vi "Begin.vi"(8 "error in":errorcluster) -> (0 "error out":errorcluster)   [LabVIEW 2015]
doc: "Called before other user functions, this VI is expected to open initial I/O refnums, load in file data, and do all program initialization. Notice that the <B>error out</B> terminal is simply used for data flow. Wiring it to other structures or subVIs ensures that this VI runs first."
uses:
  <vilib>/Rock Robotics/SystemInterfaces/DIO/FPGA_DIOPWMChannel.ctl
  <vilib>/Rock Robotics/WPI/SafetyOutput/WPI_SafetyOutputConfigMenu.ctl
  <vilib>/Rock Robotics/WPI/DriverStation/WPI_DriverStationRobotMode2.ctl
  <vilib>/Rock Robotics/WPI/Joystick/WPI_JoystickDeviceEnum.ctl
  <vilib>/Rock Robotics/WPI/Solenoid/WPI_SolenoidChannel.ctl
  <vilib>/Rock Robotics/SystemInterfaces/spilib/spi_bus.ctl
  <vilib>/Rock Robotics/SystemInterfaces/DIO/FPGA_DIOChannel.ctl
  <vilib>/Rock Robotics/WPI/RobotDrive/WPI_RobotDriveOpen2MotorWithVictor.vi
  Robot Global Data.vi
  <vilib>/Rock Robotics/Network Tables/NT Write String Array.vi
  <vilib>/Rock Robotics/WPI/MotorControl/WPI_MotorControlOpen Talon.vi
  <vilib>/Rock Robotics/WPI/Solenoid/WPI_SolenoidOpenDouble.vi
  <vilib>/Rock Robotics/WPI/Gyro/WPI_GyroXRS450_SPI_Open.vi
  <vilib>/Rock Robotics/WPI/MotorControl/WPI_MotorControlOpen Victor.vi
  <vilib>/Rock Robotics/WPI/Accelerometer/InternalAccelerometer/WPI_AccelerometerInternalOpen.vi
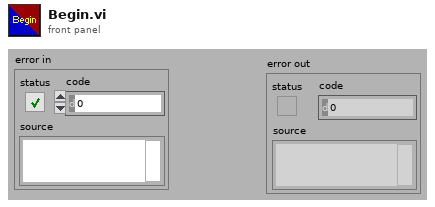
[diagram p1: front panel]
types:
  T1 = typedef "WPI_JoystickDeviceEnum.ctl" = enum16{"USB 0", "USB 1", "USB 2", "USB 3", "USB 4", "USB 5"}
  T2 = typedef "FPGA_DIOChannel.ctl" = enum8{"DIO 0", "DIO 1", "DIO 2", "DIO 3", "DIO 4", "DIO 5", "DIO 6", "DIO 7", "DIO 8", "DIO 9", "DIO MXP 0", "DIO MXP 1", "DIO MXP 2", "DIO MXP 3", "DIO MXP 4", "DIO MXP 5", "DIO MXP 6", "DIO MXP 7", "DIO MXP 8", "DIO MXP 9", "DIO MXP 10", "DIO MXP 11", "DIO MXP 12", "DIO MXP 13", "DIO MXP 14", "DIO MXP 15", "Invalid"}
  T3 = typedef "FPGA_DIOPWMChannel.ctl" = enum8{"PWM 0", "PWM 1", "PWM 2", "PWM 3", "PWM 4", "PWM 5", "PWM 6", "PWM 7", "PWM 8", "PWM 9", "PWM MXP 0", "PWM MXP 1", "PWM MXP 2", "PWM MXP 3", "PWM MXP 4", "PWM MXP 5", "PWM MXP 6", "PWM MXP 7", "PWM MXP 8", "PWM MXP 9", "Invalid"}
  T4 = typedef "WPI_SolenoidChannel.ctl" = enum8{"Solenoid 0", "Solenoid 1", "Solenoid 2", "Solenoid 3", "Solenoid 4", "Solenoid 5", "Solenoid 6", "Solenoid 7", "Invalid"}
  T5 = typedef "spi_bus.ctl" = enum16{"SPI On-Board, CS0", "SPI On-Board, CS1", "SPI On-Board, CS2", "SPI On-Board, CS3", "SPI MXP", "Invalid"}
  T6 = typedef "WPI_DriverStationRobotMode2.ctl" = enum16{"Autonomous Disabled", "Autonomous Enabled", "Teleop Disabled", "Teleop Enabled", "Disconnected", "Finish", "Test Disabled", "Test Enabled", "Emergency Stopped"}
  T7 = typedef "WPI_SafetyOutputConfigMenu.ctl" = enum16{"Enable", "Disable"}
  T8 = typedef "WPI_MotorControlDeviceRef.ctl" = cluster{"DeviceStatus":errorcluster, "Type":T9, "PWM":cluster{"PWM Channel":T3, "DeadBand":T10}, "CAN":cluster{"Device Number":u8, "Control Mode":T11, "Semaphore":T12, "Max Vout":dbl, "TalonSRX Control Mode":T13}, "Invert":bool}
  T9 = typedef "WPI_MotorControlType.ctl" = enum16{"PWM", "CAN", "CANTalonSRX"}
  T10 = typedef "WPI_PWMDeadband.ctl" = cluster{"Name":string, "maxPositivePwm":i32, "minPositivePwm":i32, "centerPwm":i32, "maxNegativePwm":i32, "minNegativePwm":i32, "angularRange":u16}
  T11 = typedef "WPI_CANJaguar_ControlMode.ctl" = enum8{"Percent VBus", "Current", "Speed", "Position", "Voltage"}
  T12 = typedef "Semaphore RefNum" = refnum<k1>
  T13 = typedef "WPI_CANTalonSRX_APIControlMode.ctl" = enum8{"Percent VBus", "Speed", "Position", "Slave", "Unchanged / Invalid", "Voltage Compensation", "Current", "Motion Profile"}
  T14 = typedef "WPI_JoystickDevRef.ctl" = cluster{"Device":T1}
  T15 = typedef "WPI_DigitalInputDevRef.ctl" = cluster{"DevStatus":errorcluster, "DIO Channel":T2}
  T16 = typedef "WPI_SolenoidDevRef.ctl" = cluster{"DevStatus":errorcluster, "Pneumatics Control Module":u8, "Forward Solenoid Channel":T4, "Reverse Solenoid Channel":T4}
  T17 = typedef "WPI_RobotDriveDevRef.ctl" = cluster{"DevStatus":errorcluster, "Motors[]":T8[], "Square Inputs":bool, "Max Output":dbl}
  T18 = typedef "WPI_GyroDevRef.ctl" = cluster{"DevStatus":errorcluster, "Analog Channel":T19, "Offset":dbl, "Gain (VoltsPerDegree/Second)":dbl, "Gyro Type":enum16{"Analog", "XRS450"}, "Handle":i32, "SPI Bus":T5, "Device Found":bool, "Sample Rate":dbl, "Calibrate On Open":bool}
  T19 = typedef "FPGA_AIChannel.ctl" = enum8{"AI 0", "AI 1", "AI 2", "AI 3", "AI MXP 0", "AI MXP 1", "AI MXP 2", "AI MXP 3", "Invalid"}
  T20 = typedef "WPI_AccelerometerDevRef.ctl" = cluster{"DevStatus":errorcluster, "Scaling":T21, "Analog Channels":T22, "I2C Bus":T23, "SPI Bus":T5, "Accel Range":T24, "ADXL Axes":T25, "Handle":i32, "Device Address":u8, "Accel Type":enum16{"Analog", "ADXL345 I2C", "ADXL345 SPI", "Internal", "ADXL362 SPI"}}
  T21 = typedef "WPI_AccelerometerScaling.ctl" = cluster{"Gain (VoltsPerG)":dbl, "Center Voltage":dbl}
  T22 = typedef "WPI_AccelerometerAnalogChannels.ctl" = cluster{"X-Axis":T19, "Y-Axis":T19, "Z-Axis":T19}
  T23 = typedef "i2c_bus.ctl" = enum16{"I2C On-Board", "I2C MXP", "Invalid"}
  T24 = typedef "ADXL345 Range.ctl" = u8
  T25 = typedef "WPI_AccelerometerADXL345 Axes.ctl" = cluster{"X-Axis":bool, "Y-Axis":bool, "Z-Axis":bool}
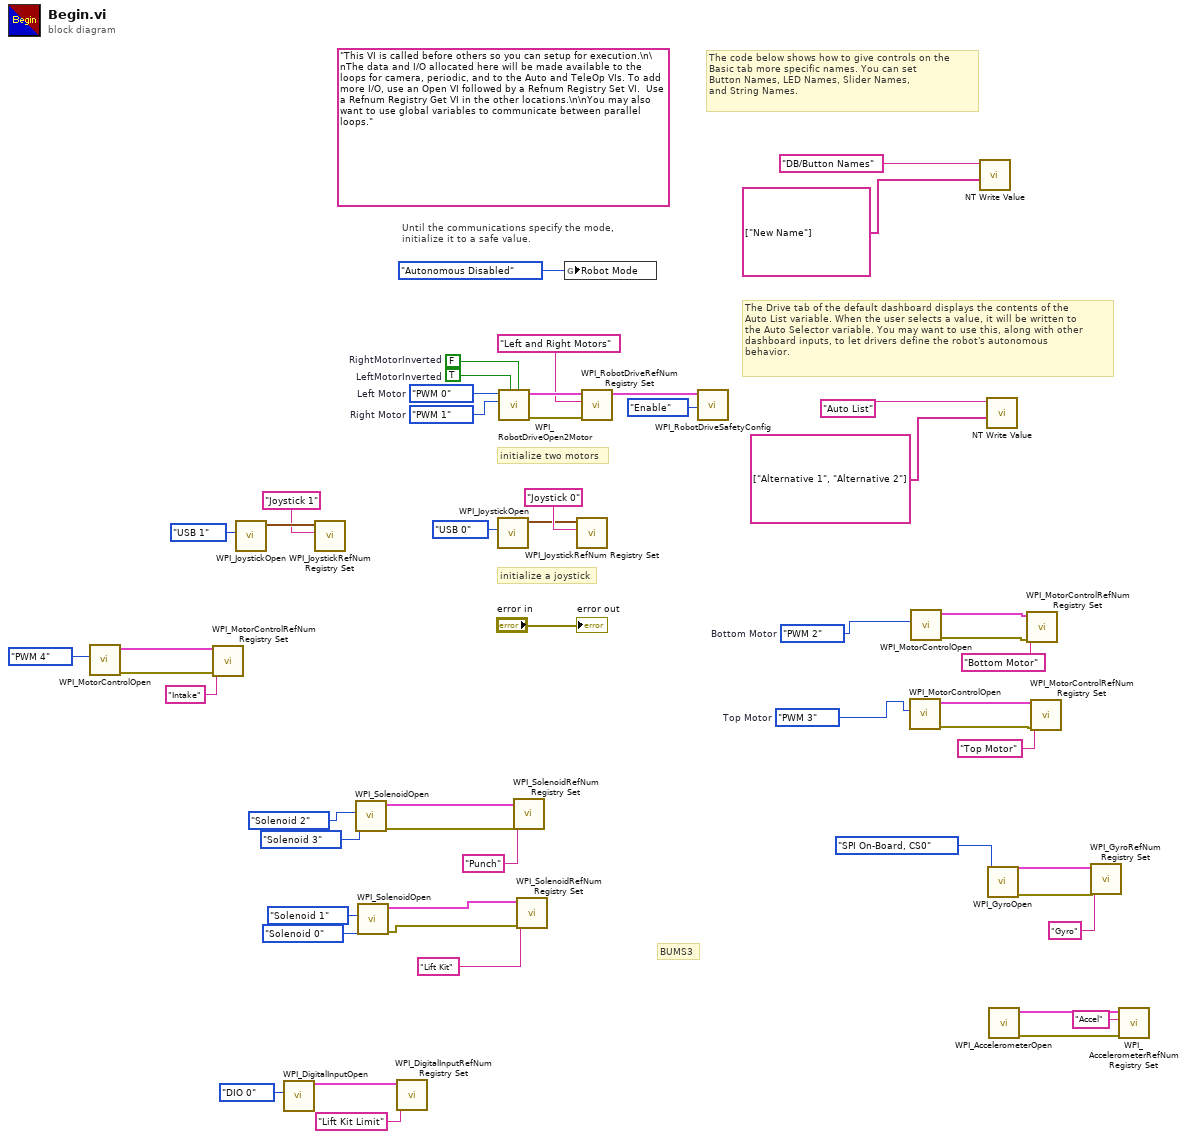
[diagram p0: block diagram]
diagram:
  w34 = FPGA_DIOPWMChannel."PWM 3"  # Top Motor
  w35 = FPGA_DIOPWMChannel."PWM 2"  # Bottom Motor
  (unwired) "This VI is called before others so you can setup for execution.\n\nThe data and I/O allocated here will be made available to the loops for camera, periodic, and to the Auto and TeleOp VIs. To add more I/O, use an Open VI followed by a Refnum Registry Set VI.  Use a Refnum Registry Get VI in the other locations.\n\nYou may also want to use global variables to communicate between parallel loops."
  w47 = FPGA_DIOPWMChannel."PWM 1"  # Right Motor
  w48 = FPGA_DIOPWMChannel."PWM 0"  # Left Motor
  w52 = TRUE  # LeftMotorInverted
  w53 = FALSE  # RightMotorInverted
  # "BUMS3"
  # "The Drive tab of the default dashboard displays the contents of the\nAuto List variable. When the user selects a value, it will be written to\nthe Auto Selector variable. You may want to use this, along with other\ndashboard inputs, to let drivers define the robot's autonomous\nbehavior."
  # "The code below shows how to give controls on the\nBasic tab more specific names. You can set\nButton Names, LED Names, Slider Names,\nand String Names."
  # "initialize a joystick"
  # "Until the communications specify the mode,\ninitialize it to a safe value."
  # "initialize two motors"
  n1 = call-poly <vilib>:"WPI_MotorControlOpen.vi"("PWM Channel"=FPGA_DIOPWMChannel."PWM 4") -> ("error out"=w8:errorcluster, "MotorControlDeviceRef"=w11:T8)  [unwired: 9 in]
  n2 = call <vilib>:"WPI_MotorControlRefNum Registry Set.vi"("error in (no error)"=w8, "refnum name"="Intake", "MotorControlDevRef"=w11) -> ()  [unwired: 7 in, 2 out]
  n3 = call <vilib>:"WPI_JoystickOpen.vi"("JoystickDevice"=WPI_JoystickDeviceEnum."USB 1") -> ("JoystickDevRef"=w2:T14)  [unwired: 10 in]
  n4 = call <vilib>:"WPI_DigitalInputOpen.vi"("DIO Channel"=FPGA_DIOChannel."DIO 0") -> ("DigitalInputDevRef"=w6:T15)  [unwired: 9 in, 1 out]
  n5 = call <vilib>:"WPI_JoystickRefNum Registry Set.vi"("refnum name"="Joystick 1", "JoystickDevRef"=w2) -> ()  [unwired: 8 in, 2 out]
  n6 = call-poly <vilib>:"WPI_SolenoidOpen.vi"("Reverse Solenoid Channel"=WPI_SolenoidChannel."Solenoid 3", "Forward Solenoid Channel"=WPI_SolenoidChannel."Solenoid 2" ("Solenoid Channel")) -> ("error out"=w7:errorcluster, "SolenoidDevRef"=w14:T16)  [unwired: 8 in]
  n7 = call-poly <vilib>:"WPI_SolenoidOpen.vi"("Reverse Solenoid Channel"=WPI_SolenoidChannel."Solenoid 0", "Forward Solenoid Channel"=WPI_SolenoidChannel."Solenoid 1" ("Solenoid Channel")) -> ("error out"=w24:errorcluster, "SolenoidDevRef"=w27:T16)  [unwired: 8 in]
  n8 = call <vilib>:"WPI_DigitalInputRefNum Registry Set.vi"("refnum name"="Lift Kit Limit", "DigitalInputDevRef"=w6) -> ()  [unwired: 8 in, 2 out]
  n9 = call <vilib>:"WPI_JoystickOpen.vi"("JoystickDevice"=WPI_JoystickDeviceEnum."USB 0") -> ("JoystickDevRef"=w42:T14)  [unwired: 10 in]
  n10 = call-poly <vilib>:"WPI_RobotDriveOpen2Motor.vi"("Right Motor Inverted"=w53, "Left Motor Inverted"=w52, "Right Motor"=w47, "Left Motor"=w48) -> ("error out"=w49:errorcluster, "RobotDriveDevRef"=w51:T17)  [unwired: 1 in, 5 out]
  n11 = call <vilib>:"WPI_SolenoidRefNum Registry Set.vi"("error in (no error)"=w7, "refnum name"="Punch", "SolenoidDevRef"=w14) -> ()  [unwired: 7 in, 2 out]
  n12 = call <vilib>:"WPI_SolenoidRefNum Registry Set.vi"("error in (no error)"=w24, "refnum name"="Lift Kit", "SolenoidDevRef"=w27) -> ()  [unwired: 7 in, 2 out]
  n13 = global write "Robot Global Data.vi" "Robot Mode"(WPI_DriverStationRobotMode2."Autonomous Disabled" ("Robot Mode")) -> ()
  n14 = call <vilib>:"WPI_JoystickRefNum Registry Set.vi"("refnum name"="Joystick 0", "JoystickDevRef"=w42) -> ()  [unwired: 8 in, 2 out]
  n15 = call <vilib>:"WPI_RobotDriveRefNum Registry Set.vi"("error in (no error)"=w49, "refnum name"="Left and Right Motors", "RobotDriveDevRef"=w51) -> ("RobotDriveDevRef"=w46:T17)  [unwired: 1 in, 7 out]
  n16 = call <vilib>:"WPI_RobotDriveSafetyConfig.vi"("mode"=WPI_SafetyOutputConfigMenu."Enable", "RobotDriveDevRef"=w46) -> ()  [unwired: 8 in, 2 out]
  n17 = call-poly <vilib>:"WPI_MotorControlOpen.vi"("PWM Channel"=w34) -> ("error out"=w28:errorcluster, "MotorControlDeviceRef"=w33:T8)  [unwired: 9 in]
  n18 = call-poly <vilib>:"WPI_MotorControlOpen.vi"("PWM Channel"=w35) -> ("error out"=w29:errorcluster, "MotorControlDeviceRef"=w32:T8)  [unwired: 9 in]
  n19 = call-poly <vilib>:"NT Write Value.vi"("String Array"=string[] ["New Name"], "Name"="DB/Button Names") -> ()  [unwired: 9 in, 1 out]
  n20 = call-poly <vilib>:"NT Write Value.vi"("String Array"=string[] ["Alternative 1", "Alternative 2"], "Name"="Auto List") -> ()  [unwired: 9 in, 1 out]
  n21 = call-poly <vilib>:"WPI_GyroOpen.vi"("SPI Bus"=spi_bus."SPI On-Board, CS0") -> ("error out"=w18:errorcluster, "GyroDevRef"=w21:T18)  [unwired: 9 in]
  n22 = call-poly <vilib>:"WPI_AccelerometerOpen.vi"() -> ("error out"=w16:errorcluster, "AccelerometerDevRef"=w19:T20)  [unwired: 10 in]
  n23 = call <vilib>:"WPI_MotorControlRefNum Registry Set.vi"("error in (no error)"=w29, "refnum name"="Bottom Motor", "MotorControlDevRef"=w32) -> ()  [unwired: 7 in, 2 out]
  n24 = call <vilib>:"WPI_MotorControlRefNum Registry Set.vi"("error in (no error)"=w28, "refnum name"="Top Motor", "MotorControlDevRef"=w33) -> ()  [unwired: 7 in, 2 out]
  n25 = call <vilib>:"WPI_GyroRefNum Registry Set.vi"("error in (no error)"=w18, "refnum name"="Gyro", "GyroDevRef"=w21) -> ()  [unwired: 7 in, 2 out]
  n26 = call <vilib>:"WPI_AccelerometerRefNum Registry Set.vi"("error in (no error)"=w16, "refnum name"="Accel", "AccelerometerDevRef"=w19) -> ()  [unwired: 7 in, 2 out]
  "error out" <- "error in"
